vi "main.vi"() -> ()   [LabVIEW 2010]
uses:
  common_typedefs/channels_cluster.ctl
  common_typedefs/clock_parameters_cluster.ctl
  scan_specification_cluster.ctl
  common_typedefs/DAC_voltage_cluster.ctl
  derived_values_cluster.ctl
  counter_cluster.ctl
  integration_cluster.ctl
  common_typedefs/DAC_values_cluster.ctl
  common_typedefs/DAC_channel_enable_cluster.ctl
  <vilib>/Platform/TimedLoop/XDataNode/XDataNode.xnode
  <vilib>/Platform/TimedLoop/XDataNode/timing_clust.ctl
  <vilib>/Platform/TimedLoop/XDataNode/nitl_modes.ctl
  <vilib>/Platform/TimedLoop/XDataNode/wakeup.ctl
  <vilib>/eio/EIONode/EIONode.xnode
  <vilib>/rvi/eio/nirviEIOImplementation/nirviEIOImplementation.xnode
  <vilib>/rvi/eio/common/nirviEmuClasses.ctl
  <vilib>/rvi/eio/common/nirviEmuTemplateMethod_noerrors.vi
  <vilib>/Platform/TimedLoop/XDataNode/XDNodeRunTimeDep.lvlib
panel:
  out "clocking":bool
  in  "clocking-trigger":bool
  out "transferred z/intensity tuples":u32
  in  "transfer z-points?":bool
  in  "invert channels":bool[](array[boolean])=[FALSE, FALSE]
  in  "enable fly-back reversion?":bool=TRUE
  in  "sync minimum high":i16=1000
  out "pixels acquired":u64
  out "counter cluster out":T1
  out "derived values":T2
  out "acquire?":bool
  in  "ADC clock phase":u8=2
  out "DAC voltages":T3 {"z-drive out" max=4095 step=1; "ch6" max=4095 step=1; "ch5" max=4095 step=1; "ch4" max=4095 step=1; "ch3" max=4095 step=1; "ch2" max=4095 step=1; "ch1" max=4095 step=1; "ch0" max=4095 step=1}
  in  "scan specification":T4={"x amplitude"=1000, "x resolution (pixels)"=200, "x offset fly-forward (iterations)"=0, "x offset fly-back (iterations)"=0, "y resolution (nr. of lines)"=200, "y step size"=5, "iterations per pixel"=5, "number of frames"=-1, "y offset (pixels)"=0, "number of y-brake lines  (before y-fly-back)"=2, "number y-brake lines (after y-fly-back)"=2, "number of y-fly-back steps"=2, "lines per z step"=0, "number of z/intensity tuples"=0}
  in  "sync?":bool
  out "clock 1 state":bool
  out "clock 2 state":bool
  out "clock 3 state":bool
  in  "clock 2 settings":T5
  in  "clock 1 settings":T5
  in  "clock 3 settings":T5
  out "data read":T6
  in  "maximum bit depth":i8
  out "FIFO overflow":bool
  in  "channel offsets":T6
  in  "scan":bool
  in  "stop":bool
  in  "wait for trigger?":bool
  in  "stop acquisition at\nFIFO overflow?":bool=TRUE
  out "scanning?":bool
  in  "converter box version":i16=2 min=1 max=2
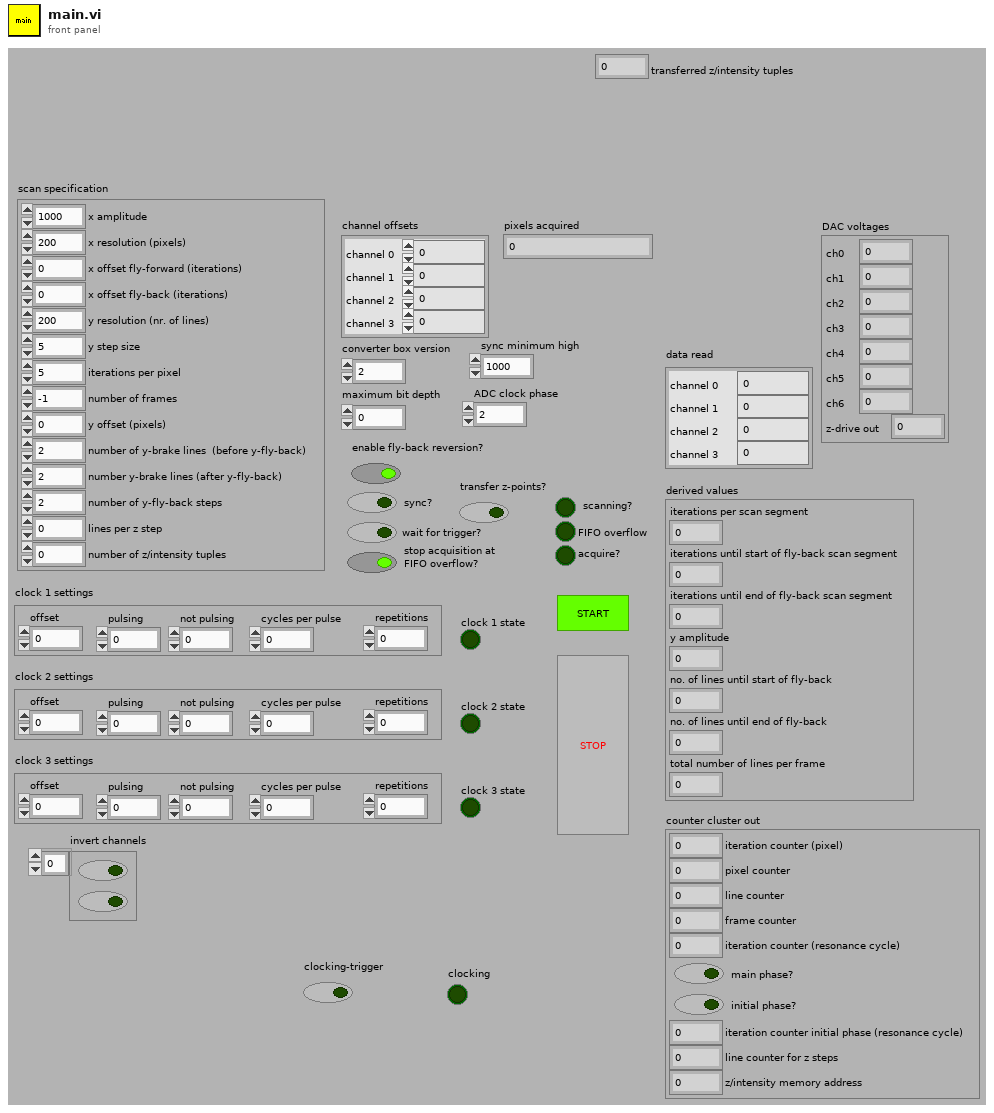
[diagram p1: front panel]
types:
  T1 = typedef "counter_cluster.ctl" = cluster{"iteration counter (pixel)":u16, "pixel counter":u16, "line counter":u16, "frame counter":u16, "iteration counter (resonance cycle)":u16, "main phase?":bool, "initial phase?":bool, "iteration counter initial phase (resonance cycle)":u16, "line counter for z steps":u16, "z/intensity memory address":u32}
  T2 = typedef "derived_values_cluster.ctl" = cluster{"iterations per scan segment":u16, "iterations until start of fly-back scan segment":u16, "iterations until end of fly-back scan segment":u16, "y amplitude":u16, "no. of lines until start of fly-back":u16, "no. of lines until end of fly-back":u16, "total number of lines per frame ":u16}
  T3 = typedef "DAC_voltage_cluster.ctl" = cluster{"ch0":u16, "ch1":u16, "ch2":u16, "ch3":u16, "ch4":u16, "ch5":u16, "ch6":u16, "z-drive out":u16}
  T4 = typedef "scan_specification_cluster.ctl" = cluster{"x amplitude":u16, "x resolution (pixels)":u16, "x offset fly-forward (iterations)":u16, "x offset fly-back (iterations)":u16, "y resolution (nr. of lines)":u16, "y step size":u16, "iterations per pixel":u16, "number of frames":i32, "y offset (pixels)":u16, "number of y-brake lines  (before y-fly-back)":u16, "number y-brake lines (after y-fly-back)":u16, "number of y-fly-back steps":u16, "lines per z step":u16, "number of z/intensity tuples":u16}
  T5 = typedef "clock_parameters_cluster.ctl" = cluster{"offset":i64, "pulsing":i64, "not pulsing":i64, "cycles per pulse":i64, "repetitions":i64}
  T6 = typedef "channels_cluster.ctl" = cluster{"channel 0":u32, "channel 1":u32, "channel 2":u32, "channel 3":u32}
  T7 = typedef "DAC_values_cluster.ctl" = cluster{"DAC channel enable":T8, "DAC voltage":T3, "offset":u16, "channel index":u16, "bit index":i32, "synch?":bool, "DAC clock":bool, "finished?":bool}
  T8 = typedef "DAC_channel_enable_cluster.ctl" = cluster{"ch0":bool, "ch1":bool, "ch2":bool, "ch3":bool, "ch4":bool, "ch5":bool, "ch6":bool}
  T9 = typedef "integration_cluster.ctl" = cluster{"channel 0":u32, "channel 1":u32, "fly-back heap address":u32}
  T10 = typedef "XDNodeRunTimeDep.lvlib/timing_clust.ctl" = cluster{"Expected End [f-1]":u64, "Actual End [f-1]":u64, "Finished Late? [f-1]":bool, "Expected End [i-1]":u64, "Actual End [i-1]":u64, "Finished Late? [i-1]":bool, "Expected Start [i]":u64, "Actual Start [i]":u64, "Expected Start [f]":u64, "Actual Start [f]":u64, "Source Name":string, "Structure Name":string, "Period":i64, "Deadline":i64, "Offset":i64, "Start":i64, "Priority":i32, "Timeout":i32, "Mode":T11, "Wakeup Reason":T12, "Error":errorcluster, "Source Type":string, "Secondary Source Type":string, "Global End Time":u64, "Global Start Time":u64, "Frame Duration":u64, "Iteration Duration":u64, "Assigned CPU":i32, "I/O Scan Engine Mode":u32}
  T11 = typedef "XDNodeRunTimeDep.lvlib/nitl_modes.ctl" = enum32{"No Change", "Process missed periods, maintain original phase", "Discard missed periods, maintain original phase", "Process missed periods, ignore original phase", "Discard missed periods, ignore original phase"}
  T12 = typedef "XDNodeRunTimeDep.lvlib/wakeup.ctl" = enum32{"Normal", "Aborted", "Asynchronous wakeup", "Timing source error", "Timed loop error", "Timeout"}
  T13 = typedef "nirviEmuClasses.ctl" = enum16{"IO Read", "IO Write", "Method", "Property Read", "Property Write"}
  T14 = typedef "gate_counters_cluster.ctl" = cluster{"phase iteration counter":i64, "phase repetition counter":i64, "pulse iteration counter":i64, "phase state":bool}
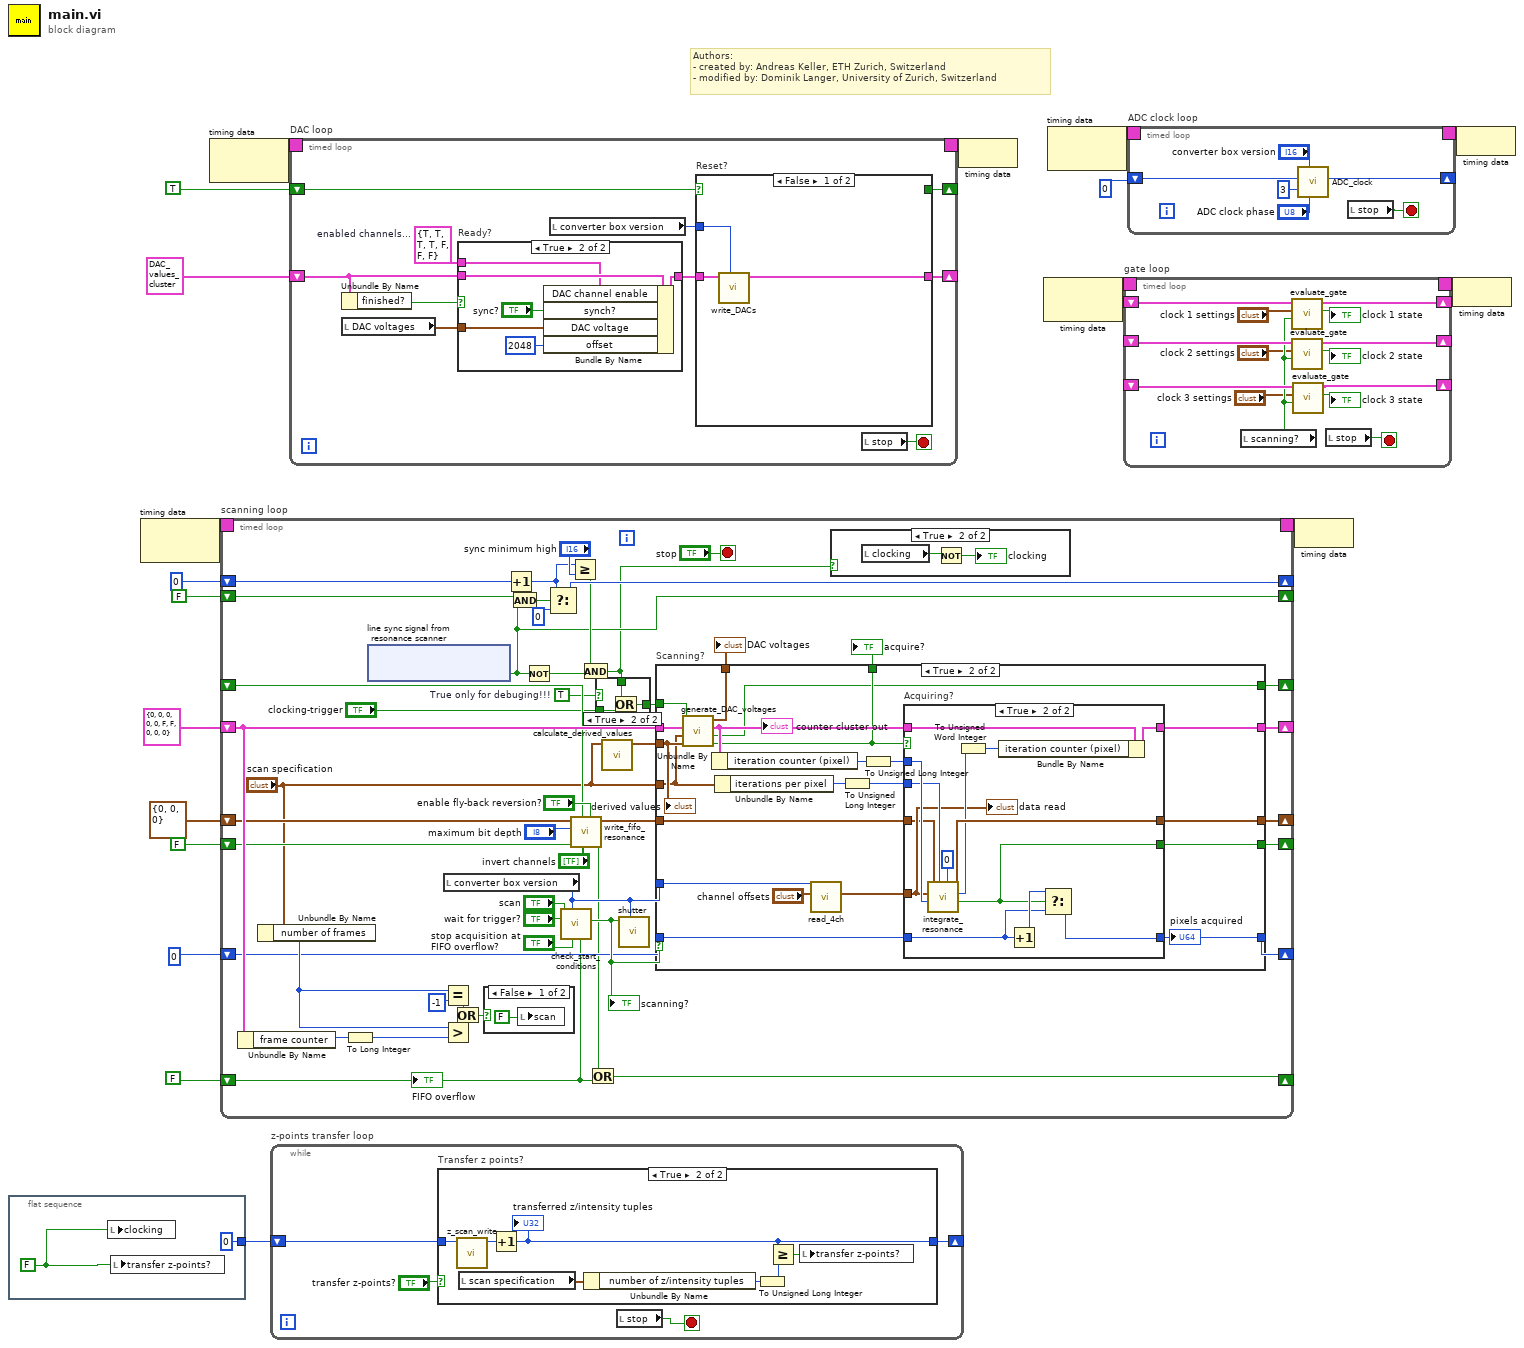
[diagram p0: block diagram]
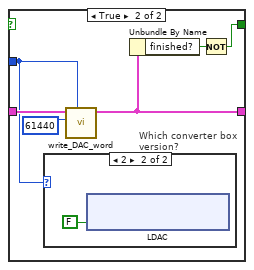
[diagram p3: hidden frame]
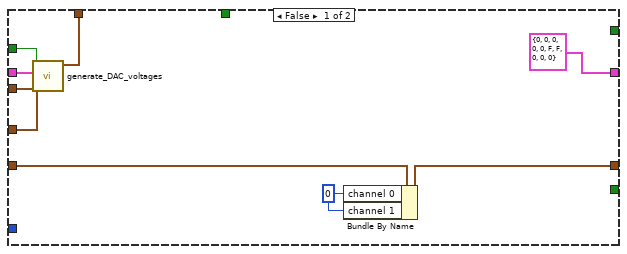
[diagram p9: hidden frame]
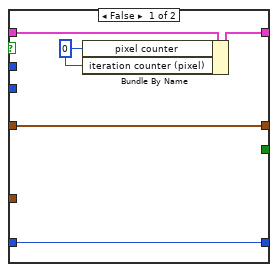
[diagram p10: hidden frame]
diagram:
  # "Authors: \n- created by: Andreas Keller, ETH Zurich, Switzerland\n- modified by: Dominik Langer, University of Zurich, Switzerland"
  n1 = flat-sequence {
    tunnel: [u32 0 ("address out")] -> w1
    frame #0 {
      w20 = FALSE ("start z-points transfer?")
      n2 = local write "clocking"(w20) -> ()
      n3 = local write "transfer z-points?"(w20) -> ()
    }
  }
  n4 = node-c288() -> (w17:T10)  [unwired: 1 in]
  n5 = node-c288() -> (w11:T10)  [unwired: 1 in]
  n6 = timed-loop "scanning loop" {
    timing: w17 -> [_]
    timing-out: [_] -> w16
    shift-right: [w67] -> _
    shift-left: T1 {"iteration counter (pixel)"=0, "pixel counter"=0, "line counter"=0, "frame counter"=0, "iteration counter (resonance cycle)"=0, "main phase?"=FALSE, "initial phase?"=FALSE, "iteration counter initial phase (resonance cycle)"=0, "line counter for z steps"=0, "z/intensity memory address"=0} ("counter cluster") -> [w57]
    shift-right: [w36] -> _
    shift-left: T9 {"channel 0"=0, "channel 1"=0, "fly-back heap address"=0} ("integration cluster") -> [w35]
    shift-right: [w38] -> _
    shift-left: FALSE -> [w29]
    shift-right: [w28] -> _
    shift-left: FALSE -> [w49]
    shift-right: [w51] -> _
    shift-left: u64 0 -> [w52]
    shift-right: [w45] -> _
    shift-left: i16 0 -> [w48]
    shift-right: [w37] -> _
    shift-left: _ -> [w33]
    shift-right: [w31] -> _
    shift-left: FALSE ("finished?") -> [w30]
    stop <- "stop" stop-if-true
    w23 = TRUE  # True only for debuging!!!
    n7 = Unbundle By Name(w57) -> ("frame counter"=w62:u16)
    n8 = Unbundle By Name("scan specification") -> ("number of frames"=w61:i32)
    n9 = To Long Integer(number=w62) -> (32bit integer=w63:i32)
    n10 = xnode "line sync signal from\nresonance scanner"() -> ("Connector0/DIO36"=w28:bool)  [unwired: 1 in, 1 out]
    n11 = Equal?(x=w61, y=-1) -> (x = y?=w55:bool)
    n12 = Greater?(x=w61, y=w63) -> (0:w64:bool)
    n13 = local read "converter box version"() -> (w60:i16)
    n14 = Or(x=w55, y=w64) -> (x .or. y?=w54:bool)
    n15 = case shown="False" w54 {
      frame False {
        n16 = local write "scan"(FALSE ("scan")) -> ()
      }
      frame True {
      }
    }
    n17 = Increment(x=w48) -> (x+1=w43:i16)
    n18 = And(x=w49, y=w28) -> (x .and. y?=w47:bool)
    n19 = Not(x=w28) -> (.not. x?=w42:bool)
    n20 = Select(t=w43, s=w47, f=i16 0) -> (s? t:f=w45:i16)
    n21 = call "check_start_conditions.vi"("FIFO overflow?"=w29, "stop at FIFO overflow?"="stop acquisition at\nFIFO overflow?", "converter box version"=w60, "in triggered mode?"="wait for trigger?", "acquire"="scan") -> ("acquire?"=w56:bool)  [unwired: 6 in]
    "scanning?" <- w56
    n22 = Greater Or Equal?(x=w43, y="sync minimum high") -> (x >= y?=w41:bool)
    n23 = call "write_fifo_resonance.vi"("enable fly-back reversion?"="enable fly-back reversion?", "invert channels"="invert channels", "fly-back?"=w33, "pixel finished?"=w30, "maximum bit depth"="maximum bit depth", "integration cluster in"=w35) -> ("FIFO overflow out"=w32:bool, "integration cluster out"=w34:T9)  [unwired: 4 in]
    n24 = And(x=w41, y=w42) -> (x .and. y?=w22:bool)
    n25 = Or(x=w32, y=w29) -> (x .or. y?=w38:bool)
    n26 = case shown="True" w23 {
      tunnel: w22 -> [w72 w75]
      tunnel: "clocking-trigger" -> [_ w74]
      tunnel: [w72 w73] -> w24
      frame False {
      }
      frame True {
        n27 = Or(x=w75, y=w74) -> (x .or. y?=w73:bool)
      }
    }
    n28 = call "calculate_derived_values.vi"("scan specification"="scan specification") -> ("derived values"=w53:T2)  [unwired: 10 in]
    n29 = call "shutter.vi"("converter box version"=w60, "open?"=w56) -> ()  [unwired: 10 in]
    n30 = case "Scanning?" shown="True" w56 {
      tunnel: w57 -> [w103 w112]
      tunnel: [T1 {"iteration counter (pixel)"=0, "pixel counter"=0, "line counter"=0, "frame counter"=0, "iteration counter (resonance cycle)"=0, "main phase?"=FALSE, "initial phase?"=FALSE, "iteration counter initial phase (resonance cycle)"=0, "line counter for z steps"=0, "z/intensity memory address"=0} ("counter cluster") w125] -> w67
      tunnel: w34 -> [w97 w120]
      tunnel: [w96 w124] -> w36
      tunnel: w60 -> [_ w119]
      tunnel: "scan specification" -> [w100 w105]
      tunnel: w24 -> [w102 w109]
      tunnel: [w101 w110] -> w58
      tunnel: w53 -> [w99 w113]
      tunnel: w52 -> [_ w115]
      tunnel: [_ w114] -> w51
      tunnel: [_ w108] -> w50
      tunnel: [_ w107] -> w31
      tunnel: [_ w106] -> w37
      frame False {
        w98 = u32 0 ("channel 0")
        n31 = call "generate_DAC_voltages.vi"("derived values"=w99, "scan specification"=w100, "counter cluster in"=w103, "resonant trigger"=w102) -> ("DAC voltages"=w101:T3)  [unwired: 4 in, 3 out]
        n32 = Bundle By Name(cluster=w97, "channel 0"=w98, "channel 1"=w98) -> (w96:T9)
      }
      frame True {
        n33 = call "generate_DAC_voltages.vi"("derived values"=w113, "scan specification"=w105, "counter cluster in"=w112, "resonant trigger"=w109) -> ("acquire?"=w108:bool, "fly-back acquisition phase?"=w106:bool, "counter cluster out"=w111:T1, "DAC voltages"=w110:T3)  [unwired: 4 in]
        "counter cluster out" <- w111
        n34 = Unbundle By Name(w111) -> ("iteration counter (pixel)"=w123:u16)
        n35 = Unbundle By Name(w105) -> ("iterations per pixel"=w122:u16)
        n36 = call "read_4ch.vi"("channel offsets"="channel offsets", "converter box version"=w119) -> ("read output"=w117:T6)  [unwired: 9 in]
        n37 = To Unsigned Long Integer(number=w122) -> (unsigned 32bit integer=w116:u32)
        n38 = To Unsigned Long Integer(number=w123) -> (unsigned 32bit integer=w118:u32)
        n39 = case "Acquiring?" shown="True" w108 {
          tunnel: w111 -> [w129 w139]
          tunnel: [w130 w137] -> w125
          tunnel: [w126 w142] -> w124
          tunnel: w120 -> [w126 w135]
          tunnel: w118 -> [_ w143]
          tunnel: w117 -> [_ w138]
          tunnel: w116 -> [_ w140]
          tunnel: w115 -> [w128 w132]
          tunnel: [w128 w134] -> w114
          tunnel: [_ w131] -> w107
          frame False {
            w127 = u16 0 ("pixel counter")
            n40 = Bundle By Name(cluster=w129, "pixel counter"=w127, "iteration counter (pixel)"=w127) -> (w130:T1)
          }
          frame True {
            n41 = call "integrate_resonance.vi"("waiting iterations per pixel"=u32 0, "integration iterations per pixel"=w140, "iteration counter in"=w143, "sampling values in"=w138, "integration cluster in"=w135) -> ("finished?"=w131:bool, "iteration counter out"=w141:u32, "integration cluster out"=w142:T9)  [unwired: 4 in]
            n42 = To Unsigned Word Integer(number=w141) -> (unsigned 16bit integer=w144:u16)
            n43 = Bundle By Name(cluster=w139, "iteration counter (pixel)"=w144) -> (w137:T1)
            n44 = Increment(x=w132) -> (x+1=w133:u64)
            n45 = Select(t=w133, s=w131, f=w132) -> (s? t:f=w134:u64)
            "data read" <- w138
          }
        }
        "pixels acquired" <- w114
        "derived values" <- w113
      }
    }
    "DAC voltages" <- w58
    "acquire?" <- w50
    n46 = case shown="True" w22 {
      frame False {
      }
      frame True {
        n47 = local read "clocking"() -> (w71:bool)
        n48 = Not(x=w71) -> (.not. x?=→"clocking":bool)
      }
    }
    "FIFO overflow" <- w29
  }
  n49 = while "z-points transfer loop" {
    shift-right: [w149] -> _
    shift-left: w1 -> [w150]
    stop <- w147 stop-if-true
    n50 = case "Transfer z points?" shown="True" "transfer z-points?" {
      tunnel: w150 -> [_ w157]
      tunnel: [_ w155] -> w149
      frame False {
      }
      frame True {
        n51 = call "z_scan_write.vi"("address in"=w157) -> ("address out"=w156:u32)  [unwired: 9 in, 1 out]
        n52 = local read "scan specification"() -> (w154:T4)
        n53 = Increment(x=w156) -> (x+1=w155:u32)
        "transferred z/intensity tuples" <- w155
        n54 = Unbundle By Name(w154) -> ("number of z/intensity tuples"=w153:u16)
        n55 = To Unsigned Long Integer(number=w153) -> (unsigned 32bit integer=w152:u32)
        n56 = Greater Or Equal?(x=w155, y=w152) -> (x >= y?=w151:bool)
        n57 = local write "transfer z-points?"(w151) -> ()
      }
    }
    n58 = local read "stop"() -> (w147:bool)
  }
  n59 = timed-loop "DAC loop" {
    timing: w11 -> [_]
    timing-out: [_] -> w10
    shift-right: [w164] -> _
    shift-left: T7 {"DAC channel enable"={"ch0"=TRUE, "ch1"=TRUE, "ch2"=FALSE, "ch3"=FALSE, "ch4"=FALSE, "ch5"=FALSE, "ch6"=FALSE}, "DAC voltage"={"ch0"=0, "ch1"=0, "ch2"=0, "ch3"=0, "ch4"=0, "ch5"=0, "ch6"=0, "z-drive out"=0}, "offset"=0, "channel index"=0, "bit index"=-1, "synch?"=FALSE, "DAC clock"=FALSE, "finished?"=TRUE} ("DAQ values out") -> [w162]
    shift-right: [w160] -> _
    shift-left: TRUE -> [w161]
    stop <- w158 stop-if-true
    w166 = T8 {"ch0"=TRUE, "ch1"=TRUE, "ch2"=TRUE, "ch3"=TRUE, "ch4"=FALSE, "ch5"=FALSE, "ch6"=FALSE}  # enabled channels...
    n60 = Unbundle By Name(w162) -> ("finished?"=w167:bool)
    n61 = local read "DAC voltages"() -> (w165:T3)
    n62 = case "Ready?" shown="True" w167 {
      tunnel: w166 -> [_ w194]
      tunnel: w162 -> [w189 w195]
      tunnel: [w189 w193] -> w163
      tunnel: w165 -> [_ w192]
      frame False {
      }
      frame True {
        n63 = Bundle By Name(cluster=w195, "DAC channel enable"=w194, "synch?"="sync?", "DAC voltage"=w192, "offset"=u16 2048) -> (w193:T7)
      }
    }
    n64 = local read "converter box version"() -> (w159:i16)
    n65 = case "Reset?" shown="False" w161 {
      tunnel: [w170 w174] -> w164
      tunnel: w163 -> [w169 w175]
      tunnel: [_ w172] -> w160
      tunnel: w159 -> [w168 w171]
      frame False {
        n66 = call "write_DACs.vi"("converter box version"=w168, "DAC values in"=w169) -> ("DAQ values out"=w170:T7)  [unwired: 9 in]
      }
      frame True {
        n67 = case "Which converter box version?" shown="2" w171 {
          frame Default {
          }
          frame 2 {
            n68 = xnode "LDAC"("Connector1/DIO32"=FALSE ("LDAC")) -> ()  [unwired: 1 in, 1 out]
          }
        }
        n69 = call "write_DAC_word.vi"("converter box version"=w171, "U16 data number"=u16 61440 ("number"), "DAC values in"=w175) -> ("DAC values out"=w174:T7)  [unwired: 8 in]
        n70 = Unbundle By Name(w174) -> ("finished?"=w173:bool)
        n71 = Not(x=w173) -> (.not. x?=w172:bool)
      }
    }
    n72 = local read "stop"() -> (w158:bool)
  }
  n73 = node-c288(w10) -> ()
  n74 = node-c288() -> (w19:T10)  [unwired: 1 in]
  n75 = node-c288() -> (w4:T10)  [unwired: 1 out]
  n76 = timed-loop "gate loop" {
    timing: w19 -> [_]
    timing-out: [_] -> w18
    shift-right: [w210] -> _
    shift-left: _ -> [w211]
    shift-right: [w207] -> _
    shift-left: _ -> [w206]
    shift-right: [w208] -> _
    shift-left: _ -> [w205]
    stop <- w209 stop-if-true
    n77 = local read "scanning?"() -> (w204:bool)
    n78 = call "evaluate_gate.vi"("acquiring?"=w204, "gate settings"="clock 1 settings", "gate counters in"=w211) -> ("pulse state out"=→"clock 1 state":bool, "gate counters out"=w210:T14)  [unwired: 7 in]
    n79 = call "evaluate_gate.vi"("acquiring?"=w204, "gate settings"="clock 2 settings", "gate counters in"=w206) -> ("pulse state out"=→"clock 2 state":bool, "gate counters out"=w207:T14)  [unwired: 7 in]
    n80 = call "evaluate_gate.vi"("acquiring?"=w204, "gate settings"="clock 3 settings", "gate counters in"=w205) -> ("pulse state out"=→"clock 3 state":bool, "gate counters out"=w208:T14)  [unwired: 7 in]
    n81 = local read "stop"() -> (w209:bool)
  }
  n82 = timed-loop "ADC clock loop" {
    timing: w4 -> [_]
    timing-out: [_] -> w3
    shift-right: [w215] -> _
    shift-left: u8 0 -> [w216]
    stop <- w218 stop-if-true
    n83 = call "ADC_clock.vi"("phase"="ADC clock phase", "converter box version"="converter box version", "iterations per cycle"=u8 3, "counter in"=w216) -> ("counter out"=w215:u8)  [unwired: 7 in]
    n84 = local read "stop"() -> (w218:bool)
  }
  n85 = node-c288(w16) -> ()
  n86 = node-c288(w18) -> ()
  n87 = node-c288(w3) -> ()
